vi "Read connection str.vi"(8 "error in":errorcluster, 11 "SharedVariableWrapper in":refnum<class "SharedVariableWrapper.lvclass">) -> (0 "error out":errorcluster, 2 "connection str":string)   [LabVIEW 2019, in "SharedVariableWrapper.lvclass"]
uses:
  SharedVariableWrapper.lvclass
  SharedVariableWrapper.lvclass/SharedVariableWrapper.ctl
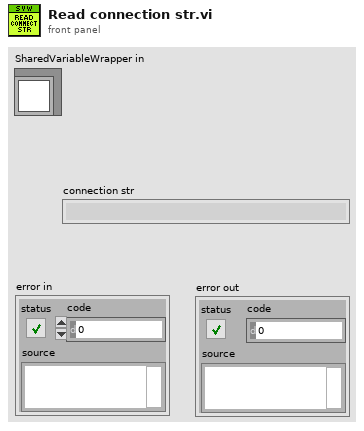
[diagram p1: front panel]
types:
  T1 = typedef "SharedVariableWrapper.lvclass/Config.ctl" = cluster{"connection str":string, "timeout":dbl, "ip":string}
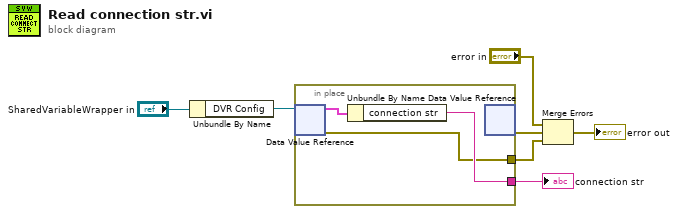
[diagram p0: block diagram]
diagram:
  n1 = Unbundle By Name("SharedVariableWrapper in") -> ("DVR Config"=w6:refnum<data-value>)
  n2 = in-place {
    in-place-border: [w9] -> w5
    in-place-border: [w8] -> w3
    n3 = in-place-dvr #1(w6) -> (w10:T1, w8:errorcluster)
    n4 = Unbundle By Name(w10) -> ("connection str"=w9:string)
    n5 = in-place-dvr #1() -> (w4:errorcluster)  [unwired: 1 in, 1 out]
  }
  "connection str" <- w5
  n6 = Merge Errors("error in", w4, w3) -> (→"error out":errorcluster)
